vi "ProcessCompletionWaiter_Valve (SubVI).vi"(11 "VISA Refnum in":refnum<visa-resource-name>) -> ()   [LabVIEW 2020]
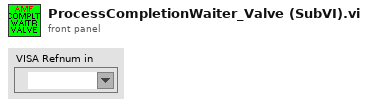
[diagram p1: front panel]
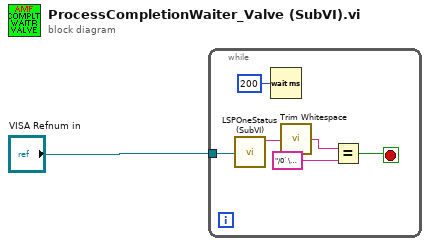
[diagram p0: block diagram]
diagram:
  n1 = while {
    tunnel: "VISA Refnum in" -> [w7]
    stop <- w6 stop-if-true
    n2 = call "LSPOneStatus (SubVI).vi"("VISA Refnum in"=w7) -> ("read buffer"=w4:string)  [unwired: 10 in]
    n3 = Wait (ms)(milliseconds to wait=u32 200) -> ()  [unwired: 1 out]
    n4 = call <vilib>:"Trim Whitespace.vi"("string"=w4) -> ("trimmed string"=w3:string)  [unwired: 1 in]
    n5 = Equal?(x=w3, y="/0`\u0003") -> (x = y?=w6:bool)
  }
